vi "Send Server Stats.vi"(8 "error in (no error)":errorcluster, 9 "timeout ms (25000)":i32=25000, 10 "Server Stats":T1={"scan rate"=10.0, "# connections"=0, "channel settings"=[]} {"channel settings"."lower input limits" format="%.4f"; "channel settings"."upper input limits" format="%.4f"; "scan rate" format="%.2f"}, 11 "refnum in":refnum<k5>) -> (0 "error out":errorcluster, 2 "bytes written":i32, 3 "refnum out":refnum<k5>)   [LabVIEW 2012]
uses:
  Server stats.ctl
panel:
  # "Hz"
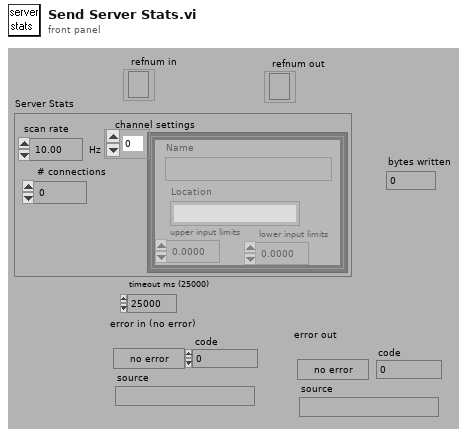
[diagram p1: front panel]
types:
  T1 = typedef "Server stats.ctl" = cluster{"scan rate":dbl, "# connections":i32, "channel settings":cluster{"Name":string, "upper input limits":sgl, "lower input limits":sgl, "Location":string}[]}
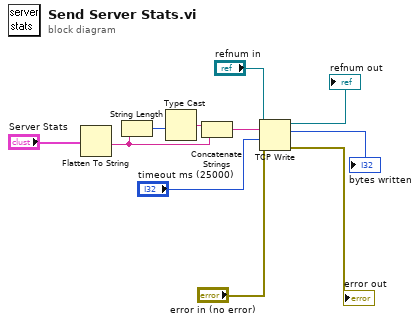
[diagram p0: block diagram]
diagram:
  n1 = Flatten To String(anything="Server Stats") -> (data string=w9:string)  [unwired: 3 in, 2 out]
  n2 = String Length(string=w9) -> (length=w3:i32)
  n3 = Type Cast(x=w3) -> (*(type *) &x=w4:string)  [unwired: 1 in]
  n4 = Concatenate Strings(w4, w9) -> (w2:string)
  n5 = TCP Write(connection ID="refnum in", data in=w2, error in (no error)="error in (no error)", 9:"timeout ms (25000)") -> (connection ID out=→"refnum out":refnum<k5>, bytes written=→"bytes written":i32, error out=→"error out":errorcluster)
